vi "Drive Controller.vi"(8 "error in":errorcluster) -> ()   [LabVIEW 2019]
doc: "This VI executes continuously carrying out the current operation and responding to updates or new operation requests. It will often contain the timing or control code that is difficult to place directly in TeleOp. This VI generally opens all sensors and motors and isolates the rest of the robot code from knowing implementation details of how the operations are carried out."
uses:
  <vilib>/Rock Robotics/WPI/Framework/Completion Status.ctl
  Drive Setpoints.ctl
  Drive Operations.ctl
  <vilib>/Rock Robotics/WPI/ThirdParty/REV Robotics/SPARK MAX/Typedef/Spark MAX Control Type.ctl
panel:
  in  "Interactive Values":T1
  in  "Buttons":cluster{"Execute Cmd":bool, "Abort Cmd":bool}
  out "Command Timing":cluster{"Start Time (ms)":u32, "Iterations":i32}
  out "Status":T3
  out "Setpoints":T4(graph)
  out "Current\nCmd":string
  # "Tip: The graph shows the motor setpoints. It may also be helpful to observe inputs and sensor values.\nYou may also want to display tuning or debugging controls."
  # "Interactive Command: You may fill in the settings for a command\nand schedule it with the Execute button. You can observe and abort\nany command while fine tuning the code for the controller."
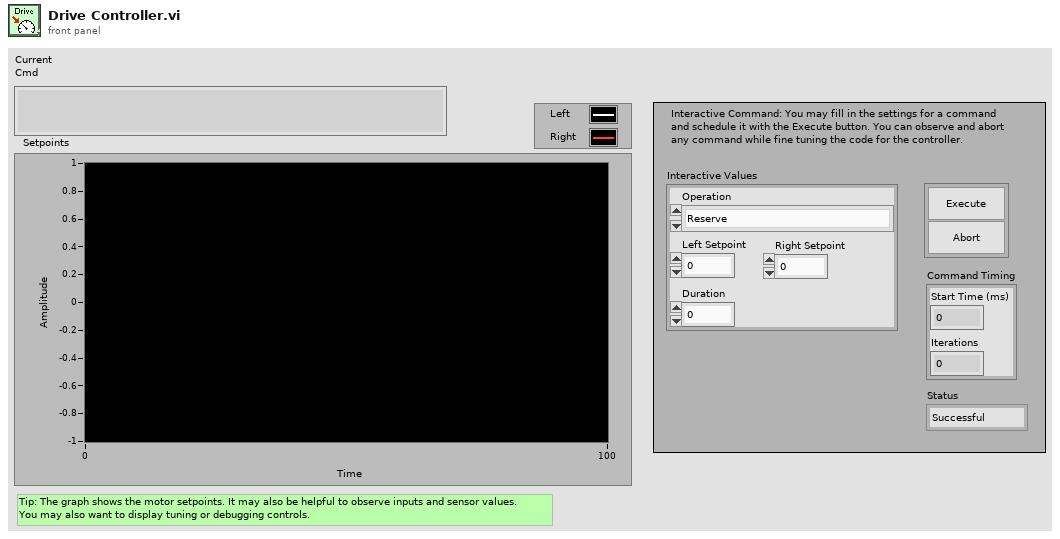
[diagram p1: front panel]
types:
  T1 = typedef "Drive Setpoints.ctl" = cluster{"Operation":T2, "Left Setpoint":dbl, "Right Setpoint":dbl, "Duration":dbl}
  T2 = typedef "Drive Operations.ctl" = enum16{"Reserve", "Read Current", "Immediate", "Drive for Time", "Drive for Distance"}
  T3 = typedef "Completion Status.ctl" = enum16{"Successful", "Aborted", "Incomplete"}
  T4 = cluster{"Left Setpoint":dbl, "Right Setpoint":dbl}
  T5 = typedef "WPI_MotorControlDeviceRef.ctl" = cluster{"DeviceStatus":errorcluster, "Type":T6, "PWM":cluster{"PWM Channel":T7, "DeadBand":T8}, "CAN":cluster{"Device Number":u8, "SetOutput VI Ref":variant, "GetOutput VI Ref":variant, "Enable VI Ref":variant, "Disable VI Ref":variant, "Data":variant}, "Invert":bool, "DIO PWM":cluster{"PWM \"Enable\" Channel":T7, "DIOChannel":T9, "PWM Rate":dbl}}
  T6 = typedef "WPI_MotorControlType.ctl" = enum16{"PWM", "CAN", "DIO PWM"}
  T7 = typedef "FPGA_DIOPWMChannel.ctl" = enum8{"PWM 0", "PWM 1", "PWM 2", "PWM 3", "PWM 4", "PWM 5", "PWM 6", "PWM 7", "PWM 8", "PWM 9", "PWM MXP 0", "PWM MXP 1", "PWM MXP 2", "PWM MXP 3", "PWM MXP 4", "PWM MXP 5", "PWM MXP 6", "PWM MXP 7", "PWM MXP 8", "PWM MXP 9", "Invalid"}
  T8 = typedef "WPI_PWMDeadband.ctl" = cluster{"Name":string, "maxPositivePwm":i32, "minPositivePwm":i32, "centerPwm":i32, "maxNegativePwm":i32, "minNegativePwm":i32, "angularRange":u16}
  T9 = typedef "FPGA_DIOChannel.ctl" = enum8{"DIO 0", "DIO 1", "DIO 2", "DIO 3", "DIO 4", "DIO 5", "DIO 6", "DIO 7", "DIO 8", "DIO 9", "DIO MXP 0", "DIO MXP 1", "DIO MXP 2", "DIO MXP 3", "DIO MXP 4", "DIO MXP 5", "DIO MXP 6", "DIO MXP 7", "DIO MXP 8", "DIO MXP 9", "DIO MXP 10", "DIO MXP 11", "DIO MXP 12", "DIO MXP 13", "DIO MXP 14", "DIO MXP 15", "SPI Port CS1", "SPI Port CS2", "SPI Port CS3", "SPI Port MISO", "SPI Port MOSI", "Invalid"}
  T10 = cluster{"MotorControlDeviceRef":T5, "error out":errorcluster, "MotorControlDeviceRef":T5, "error out":errorcluster}
  T11 = typedef "Command Status Info.ctl" = cluster{"Name":string, "Status":T3, "notifier out":T12}
  T12 = typedef "Completion Notifier.ctl" = refnum<notifier>
  T13 = cluster{"SubSystem Data":T1, cluster{"Start Time (ms)":u32, "Iterations":i32}, cluster{"Command Info":T11, "Description":string, "Default Command":T1, "queue out":refnum<queue>, "Subsystem Name":string}}
  T14 = typedef "Spark MAX Control Type.ctl" = enum16{"Percent VBus", "Voltage", "Velocity", "Position", "Smart Motion", "Current", "Smart Velocity"}
  T15 = cluster{"SubSystem Data":T1, cluster{"Start Time (ms)":u32, "Iterations":i32}, "Default Command Arguments":cluster{"Command Info":T11, "Description":string, "Default Command":T1, "queue out":refnum<queue>, "Subsystem Name":string}}
  T16 = cluster{"Don't move motors while reserved":dbl, "Don't move motors while reserved":dbl}
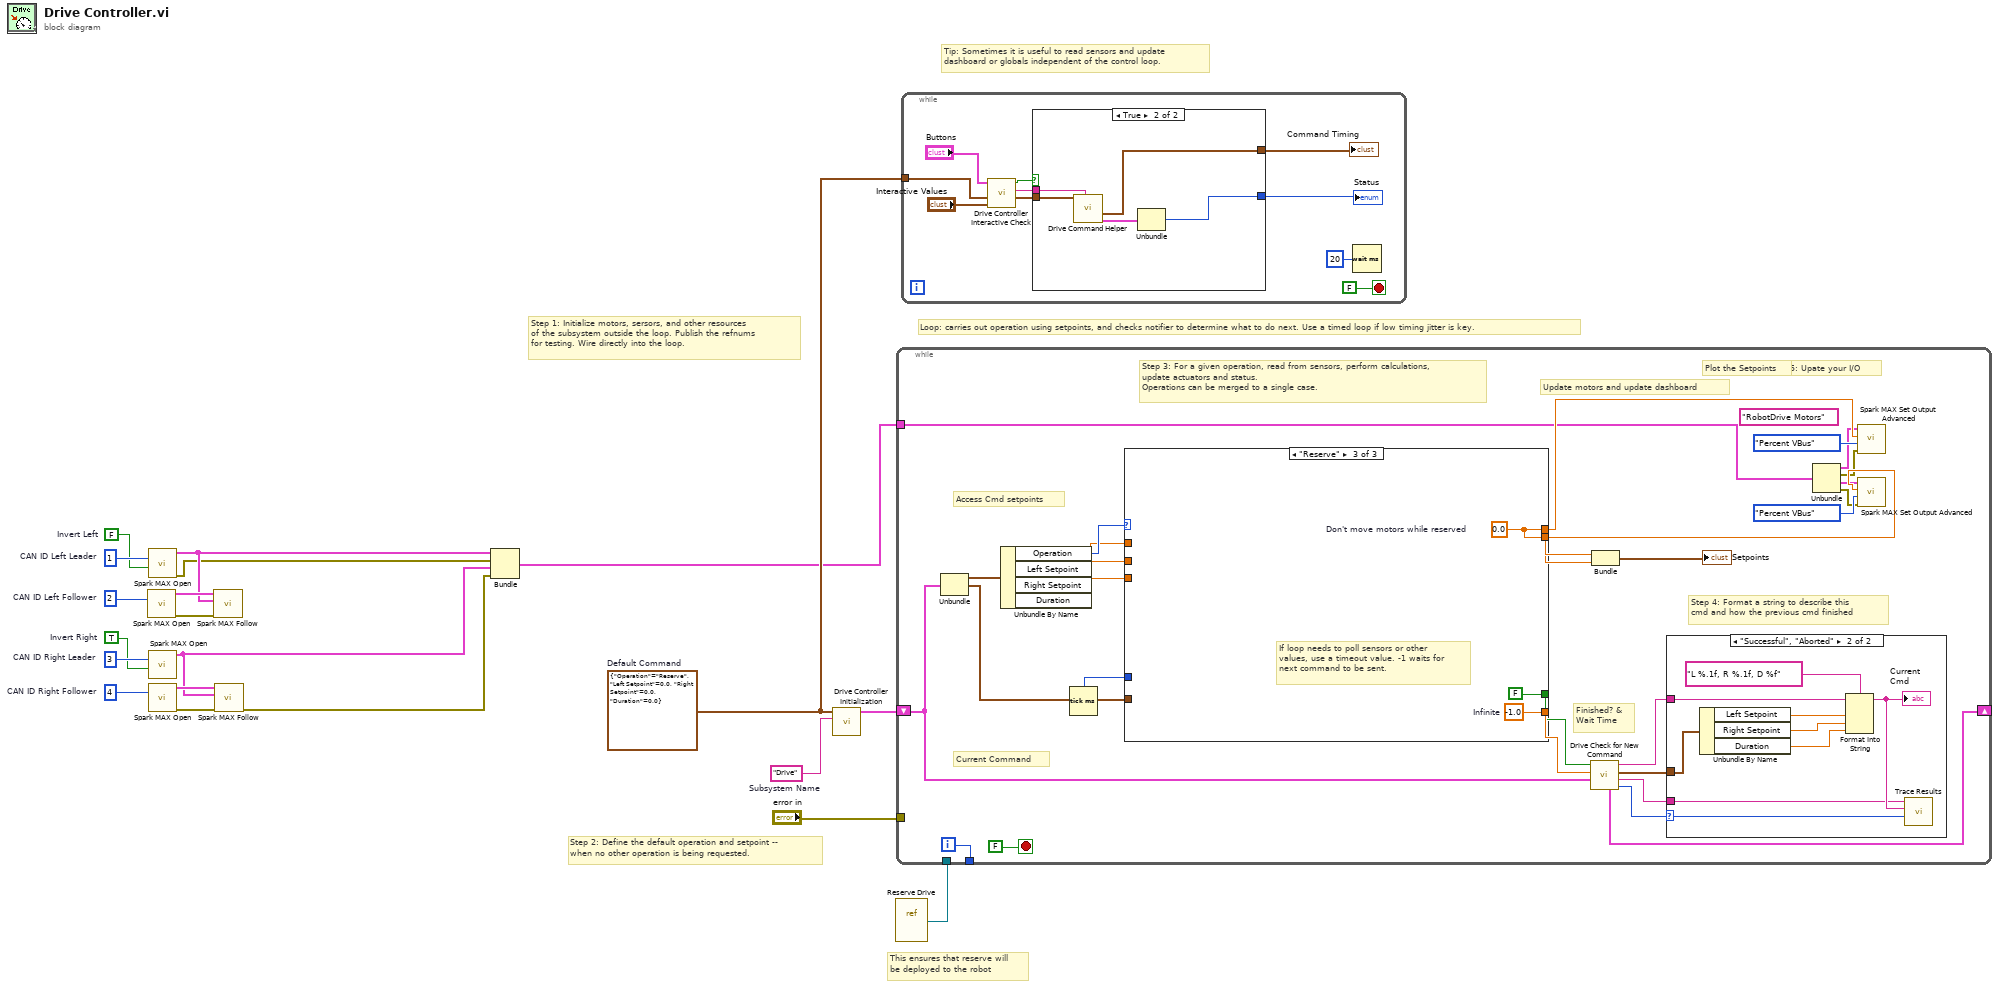
[diagram p0: block diagram]
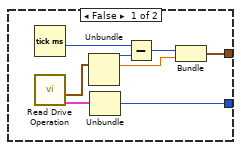
[diagram p2: hidden frame]
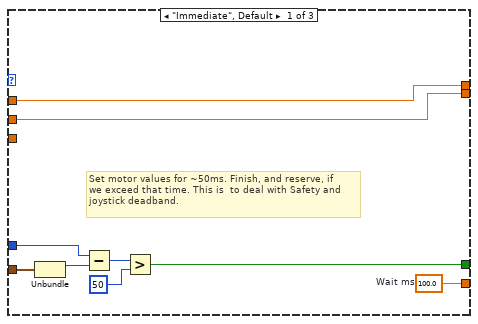
[diagram p4: hidden frame]
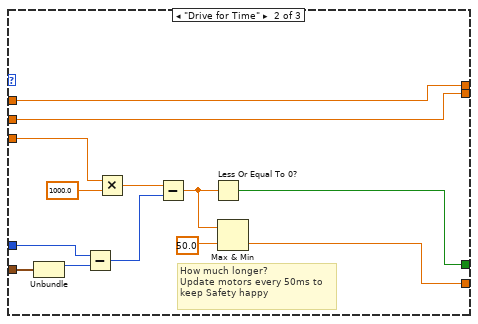
[diagram p5: hidden frame]
diagram:
  w6 = FALSE  # Invert Left
  w7 = TRUE  # Invert Right
  w9 = u8 3  # CAN ID Right Leader
  w8 = u8 4  # CAN ID Right Follower
  w14 = u8 1  # CAN ID Left Leader
  w15 = u8 2  # CAN ID Left Follower
  w16 = T1 {"Operation"=enum."Reserve", "Left Setpoint"=0.0, "Right Setpoint"=0.0, "Duration"=0.0}  # Default Command
  w20 = "Drive"  # Subsystem Name
  # "This ensures that reserve will\nbe deployed to the robot"
  # "Tip: Sometimes it is useful to read sensors and update\ndashboard or globals independent of the control loop."
  # "Step 2: Define the default operation and setpoint --\nwhen no other operation is being requested."
  # "Step 1: Initialize motors, sersors, and other resources\nof the subsystem outside the loop. Publish the refnums\nfor testing. Wire directly into the loop."
  # "Loop: carries out operation using setpoints, and checks notifier to determine what to do next. Use a timed loop if low timing jitter is key."
  n1 = call <vilib>:"Spark MAX Open.vi"("Device Number"=w15) -> ("error out"=w12:errorcluster, "MotorControlDeviceRef"=w13:T5)  [unwired: 9 in]
  n2 = call <vilib>:"Spark MAX Open.vi"("Invert"=w6, "Device Number"=w14) -> ("error out"=w3:errorcluster, "MotorControlDeviceRef"=w5:T5)  [unwired: 8 in]
  n3 = call <vilib>:"Spark MAX Open.vi"("Invert"=w7, "Device Number"=w9) -> ("MotorControlDeviceRef"=w4:T5)  [unwired: 8 in, 1 out]
  n4 = call <vilib>:"Spark MAX Open.vi"("Device Number"=w8) -> ("error out"=w11:errorcluster, "MotorControlDeviceRef"=w10:T5)  [unwired: 9 in]
  n5 = call <vilib>:"Spark MAX Follow.vi"("error in (no error)"=w12, "Master Controller"=w5, "MotorControlDeviceRef"=w13) -> ()  [unwired: 7 in, 2 out]
  n6 = call <vilib>:"Spark MAX Follow.vi"("error in (no error)"=w11, "Master Controller"=w4, "MotorControlDeviceRef"=w10) -> ("error out"=w2:errorcluster)  [unwired: 7 in, 1 out]
  n7 = Bundle("MotorControlDeviceRef"=w5, "error out"=w3, "MotorControlDeviceRef"=w4, "error out"=w2) -> (w1:T10)  [unwired: 1 in]
  n8 = call "Drive Controller Initialization.vi"("Subsystem Name"=w20, "Default Command"=w16) -> ("Current Command"=w18:T13)  [unwired: 9 in]
  n9 = vi-ref "Reserve Drive.vi"() -> (w17:refnum<vi>)
  n10 = while {
    shift-right: [w37] -> _
    shift-left: w18 -> [w30]
    tunnel: [w46] -> _
    tunnel: "error in" -> [_]
    tunnel: w17 -> [_]
    tunnel: w1 -> [w25]
    i -> [w46]
    stop <- FALSE stop-if-true
    (unwired) "RobotDrive Motors" ("Name")
    # "Step 5: Upate your I/O"
    # "Step 4: Format a string to describe this\ncmd and how the previous cmd finished"
    # "Current Command"
    # "Update motors and update dashboard"
    # "Plot the Setpoints"
    # "Access Cmd setpoints"
    # "Finished? &\nWait Time"
    # "Step 3: For a given operation, read from sensors, perform calculations,\nupdate actuators and status.\nOperations can be merged to a single case."
    n11 = Unbundle(w30) -> ("SubSystem Data"=w44:T1, w31:cluster{"Start Time (ms)":u32, "Iterations":i32})  [unwired: 1 out]
    n12 = Unbundle By Name(w44) -> ("Operation"=w43:T2, "Left Setpoint"=w42:dbl, "Right Setpoint"=w41:dbl, "Duration"=w40:dbl)
    n13 = Tick Count (ms)() -> (millisecond timer value=w39:u32)
    n14 = case shown="\"Reserve\"" w43 {
      tunnel: [w65 w66 w81] -> w36
      tunnel: [w58 w73 FALSE ("ignore previous (F)")] -> w35
      tunnel: w31 -> [w57 w75 _]
      tunnel: [w64 w72 w79] -> w27
      tunnel: [w63 w71 w79] -> w26
      tunnel: w42 -> [w64 w72 _]
      tunnel: w41 -> [w63 w71 _]
      tunnel: w40 -> [_ w70 _]
      tunnel: w39 -> [w59 w69 _]
      frame "Immediate", Default {
        w65 = 100.0  # Wait ms
        # "Set motor values for ~50ms. Finish, and reserve, if\nwe exceed that time. This is  to deal with Safety and\njoystick deadband."
        n15 = Unbundle(w57) -> ("Start Time (ms)"=w60:u32)  [unwired: 1 out]
        n16 = Subtract(x=w59, y=w60) -> (x-y=w61:u32)
        n17 = Greater?(x=w61, y=u8 50 ("Left Motor")) -> (0:w58:bool)
      }
      frame "Drive for Time" {
        # "How much longer?\nUpdate motors every 50ms to\nkeep Safety happy"
        n18 = Unbundle(w75) -> ("Start Time (ms)"=w74:u32)  [unwired: 1 out]
        n19 = Subtract(x=w69, y=w74) -> (x-y=w78:u32)
        n20 = Multiply(x=w70, y=1000.0) -> (x*y=w77:dbl)
        n21 = Subtract(x=w77, y=w78) -> (x-y=w68:dbl)
        n22 = Less Or Equal To 0?(x=w68) -> (x <= 0?=w73:bool)
        n23 = Max & Min(x=w68, y=50.0) -> (min(x,y)=w66:dbl)  [unwired: 1 out]
      }
      frame "Reserve" {
        w79 = 0.0  # Don't move motors while reserved
        w81 = -1.0  # Infinite
        # "If loop needs to poll sensors or other\nvalues, use a timeout value. -1 waits for\nnext command to be sent."
      }
    }
    n24 = call "Drive Check for New Command.vi"("input cluster"=w30, "Wait time (ms)"=w36, "Finished?"=w35) -> ("Completion"=w38:T3, "Subsystem Name"=w32:string, "Current Command"=w33:T1, "Initial Trace String"=w34:string, "Next Command"=w37:T15)  [unwired: 4 in]
    n25 = Bundle("Don't move motors while reserved"=w27, "Don't move motors while reserved"=w26) -> (→"Setpoints":T16)  [unwired: 1 in]
    n26 = case shown="\"Successful\", \"Aborted\"" w38 {
      selector: w38 -> [_ w56]
      tunnel: w34 -> [_ w51]
      tunnel: w33 -> [_ w52]
      tunnel: w32 -> [_ w48]
      frame "Incomplete", Default {
        # "Continuing current command"
      }
      frame "Successful", "Aborted" {
        # "Report and setup for next command"
        n27 = Unbundle By Name(w52) -> ("Left Setpoint"=w54:dbl, "Right Setpoint"=w55:dbl, "Duration"=w49:dbl)
        n28 = Format Into String(format string="L %.1f, R %.1f, D %f", initial string=w51, w54, w55, w49) -> (resulting string=w50:string)  [unwired: 1 in, 1 out]
        "Current\nCmd" <- w50
        n29 = call <vilib>:"Trace Results.vi"("Status of previous command"=w56, "Description"=w50, "Subsystem"=w48) -> ()  [unwired: 9 in]
      }
    }
    n30 = Unbundle(w25) -> ("MotorControlDeviceRef"=w24:T5, "error out"=w23:errorcluster, "MotorControlDeviceRef"=w22:T5, "error out"=w21:errorcluster)
    n31 = call <vilib>:"Spark MAX Set Output Advanced.vi"("error in (no error)"=w23, "Control Mode"=Spark_MAX_Control_Type."Percent VBus", "Setpoint"=w27, "MotorControlDevRef"=w24) -> ()  [unwired: 6 in, 2 out]
    n32 = call <vilib>:"Spark MAX Set Output Advanced.vi"("error in (no error)"=w21, "Control Mode"=Spark_MAX_Control_Type."Percent VBus", "Setpoint"=w26, "MotorControlDevRef"=w22) -> ()  [unwired: 6 in, 2 out]
  }
  n33 = while {
    tunnel: w16 -> [w83]
    stop <- FALSE stop-if-true
    n34 = call "Drive Controller Interactive Check.vi"("Interactive Command In"="Interactive Values", "Default Command"=w83, "Buttons"="Buttons") -> ("Interactive Command Out"=w85:T1, "Trace String"=w86:string, "Schedule"=w87:bool)  [unwired: 6 in]
    n35 = case shown="True" w87 {
      tunnel: [w96 w104] -> w88
      tunnel: [w95 w100] -> w89
      tunnel: w86 -> [_ w102]
      tunnel: w85 -> [_ w101]
      frame False {
        n36 = Tick Count (ms)() -> (millisecond timer value=w99:u32)
        n37 = call "Read Drive Operation.vi"() -> ("Command Info"=w93:T11, "SubSystem Data"=w92:T1)  [unwired: 9 in, 1 out]
        n38 = Unbundle(w92) -> ("Operation"=w97:T2, "Left Setpoint"=w94:dbl)  [unwired: 2 out]
        n39 = Unbundle(w93) -> ("Status"=w96:T3)  [unwired: 2 out]
        n40 = Subtract(x=w99, y=w97) -> (x-y=w98:u32)
        n41 = Bundle(w98, "Left Setpoint"=w94) -> (w95:cluster{u32, "Left Setpoint":dbl})  [unwired: 1 in]
      }
      frame True {
        n42 = call "Drive Command Helper.vi"("Description"=w102, "SubSystem Data"=w101) -> ("Command Info Out"=w103:T11, "Command Timing"=w100:cluster{"Start Time (ms)":u32, "Iterations":i32})  [unwired: 7 in, 1 out]
        n43 = Unbundle(w103) -> ("Status"=w104:T3)  [unwired: 2 out]
      }
    }
    "Status" <- w88
    "Command Timing" <- w89
    n44 = Wait (ms)(milliseconds to wait=u32 20) -> ()  [unwired: 1 out]
  }
